vi "ClearRebootLog.vi"(8 "error in":errorcluster, 11 "log path":path) -> (0 "error out":errorcluster)   [LabVIEW 2017, in "Controller.lvlib"]
uses:
  <vilib>/addons/InsightCM/Devices/Shared/Common/Controller/Controller.lvlib
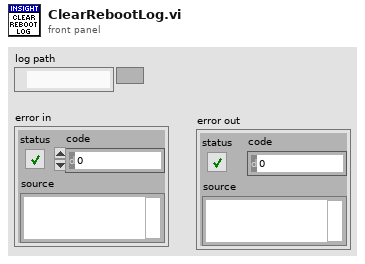
[diagram p1: front panel]
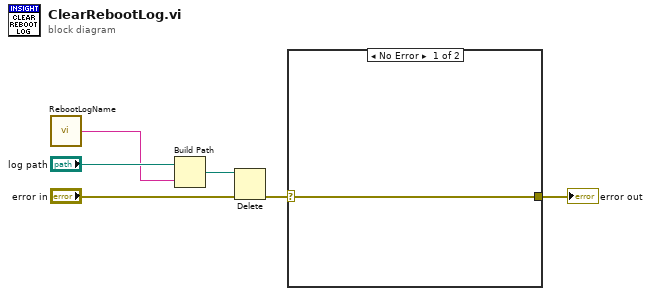
[diagram p0: block diagram]
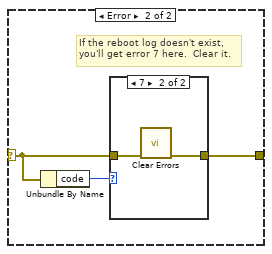
[diagram p2: hidden frame]
diagram:
  n1 = call <vilib>:"RebootLogName.vi"() -> ("reboot log name"=w4:string)  [unwired: 5 in]
  n2 = Build Path(base path="log path", name or relative path=w4) -> (appended path=w5:path)
  n3 = Delete(path (use dialog)=w5, error in="error in") -> (error out=w2:errorcluster)  [unwired: 3 in, 2 out]
  n4 = case shown="No Error" w2 {
    selector: w2 -> [w7 w9]
    tunnel: [w7 w8] -> w1
    frame No Error {
    }
    frame Error {
      # "If the reboot log doesn't exist,\nyou'll get error 7 here.  Clear it."
      n5 = Unbundle By Name(w9) -> ("code"=w10:i32)
      n6 = case shown="7" w10 {
        tunnel: w9 -> [w11 w13]
        tunnel: [w11 w12] -> w8
        frame 0, Default {
        }
        frame 7 {
          n7 = call <vilib>:"Clear Errors.vi"("error in (no error)"=w13) -> ("error out"=w12:errorcluster)  [unwired: 5 in, 1 out]
        }
      }
    }
  }
  "error out" <- w1
